vi "Rearrange images.vi"() -> ()   [LabVIEW 2015]
panel:
  in  "Selet tab":enum16{"Diagnostics", "Main"}(ring)
  in  "Type of label":u16(ring) items=["Combo", "String"]
  in  "Update\nTables":bool=TRUE
  in  "#Racks":u8
  in  "Camera names":string[](array[string])
  in  "Table column headers":string[](array[string])
  in  "Image indicator layouts 2":T1(array[cluster])=[{"NumberOfImageIndicators"=0.0, "ImageSpecificData"=[{"Width"=0.0, "Left"=0.0, "Top"=0.0, "Image Percentage"={"Height"=0.0, "Width correction"=0.0, "Height correction"=0.0, "Left correction"=0.0, "Top correction"=0.0}, "String Percentage"={"Height"=0.0, "Width correction"=0.0, "Height correction"=0.0, "Left correction"=0.0, "Top correction"=0.0}}, {"Width"=0.0, "Left"=0.0, "Top"=0.0, "Image Percentage"={"Height"=0.0, "Width correction"=0.0, "Height correction"=0.0, "Left correction"=0.0, "Top correction"=0.0}, "String Percentage"={"Height"=0.0, "Width correction"=0.0, "Height correction"=0.0, "Left correction"=0.0, "Top correction"=0.0}}, {"Width"=0.5, "Left"=0.0, "Top"=0.0, "Image Percentage"={"Height"=0.45, "Width correction"=-10.0, "Height correction"=0.0, "Left correction"=0.0, "Top correction"=0.0}, "String Percentage"={"Height"=0.05, "Width correction"=-5.0, "Height correction"=0.0, "Left correction"=0.0, "Top correction"=0.0}}, {"Width"=0.5, "Left"=0.0, "Top"=0.5, "Image Percentage"={"Height"=0.0, "Width correction"=-10.0, "Height correction"=0.0, "Left correction"=0.0, "Top correction"=0.0}, "String Percentage"={"Height"=0.0, "Width correction"=-5.0, "Height correction"=0.0, "Left correction"=0.0, "Top correction"=0.0}}, {"Width"=0.5, "Left"=0.5, "Top"=0.0, "Image Percentage"={"Height"=0.95, "Width correction"=-10.0, "Height correction"=0.0, "Left correction"=0.0, "Top correction"=0.0}, "String Percentage"={"Height"=0.05, "Width correction"=-5.0, "Height correction"=0.0, "Left correction"=0.0, "Top correction"=0.0}}]}, {"NumberOfImageIndicators"=0.0, "ImageSpecificData"=[]}, {"NumberOfImageIndicators"=0.0, "ImageSpecificData"=[{"Width"=0.5, "Left"=0.0, "Top"=0.0, "Image Percentage"={"Height"=0.45, "Width correction"=-7.0, "Height correction"=0.0, "Left correction"=0.0, "Top correction"=0.0}, "String Percentage"={"Height"=0.05, "Width correction"=-5.0, "Height correction"=0.0, "Left correction"=0.0, "Top correction"=0.0}}, {"Width"=0.5, "Left"=0.0, "Top"=0.5, "Image Percentage"={"Height"=0.45, "Width correction"=-7.0, "Height correction"=0.0, "Left correction"=0.0, "Top correction"=0.0}, "String Percentage"={"Height"=0.05, "Width correction"=-5.0, "Height correction"=0.0, "Left correction"=0.0, "Top correction"=0.0}}, {"Width"=0.5, "Left"=0.5, "Top"=0.0, "Image Percentage"={"Height"=0.95, "Width correction"=-7.0, "Height correction"=0.0, "Left correction"=0.0, "Top correction"=0.0}, "String Percentage"={"Height"=0.05, "Width correction"=-5.0, "Height correction"=0.0, "Left correction"=0.0, "Top correction"=0.0}}, {"Width"=0.5, "Left"=0.0, "Top"=0.5, "Image Percentage"={"Height"=0.45, "Width correction"=-7.0, "Height correction"=0.0, "Left correction"=0.0, "Top correction"=0.0}, "String Percentage"={"Height"=0.05, "Width correction"=-5.0, "Height correction"=0.0, "Left correction"=0.0, "Top correction"=0.0}}, {"Width"=0.5, "Left"=0.5, "Top"=0.0, "Image Percentage"={"Height"=0.0, "Width correction"=-7.0, "Height correction"=0.0, "Left correction"=0.0, "Top correction"=0.0}, "String Percentage"={"Height"=0.0, "Width correction"=-5.0, "Height correction"=0.0, "Left correction"=0.0, "Top correction"=0.0}}]}]
  in  "References":T2
  out "error out":errorcluster
  in  "error in (no error)":errorcluster
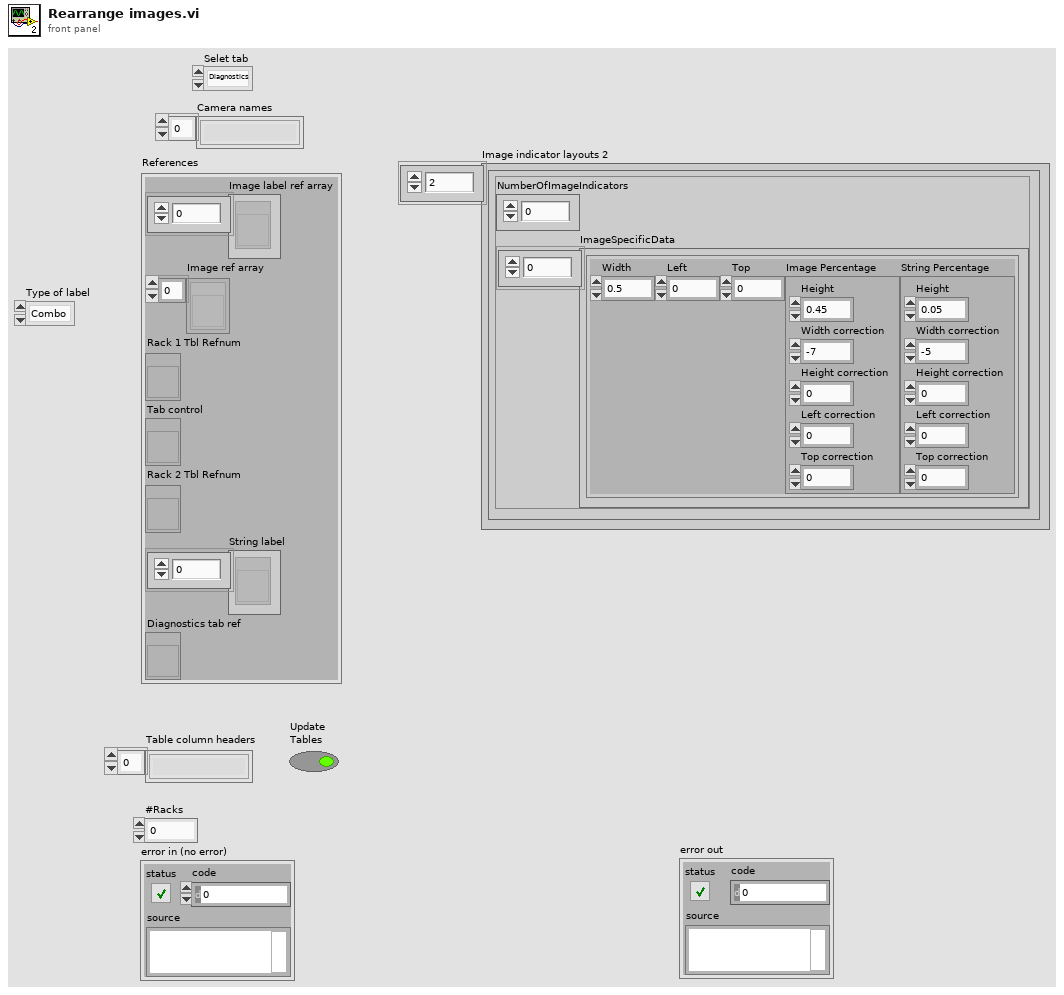
[diagram p1: front panel]
types:
  T1 = cluster{"NumberOfImageIndicators":dbl, "ImageSpecificData":cluster{"Width":dbl, "Left":dbl, "Top":dbl, "Image Percentage":cluster{"Height":dbl, "Width correction":dbl, "Height correction":dbl, "Left correction":dbl, "Top correction":dbl}, "String Percentage":cluster{"Height":dbl, "Width correction":dbl, "Height correction":dbl, "Left correction":dbl, "Top correction":dbl}}[]}[]
  T2 = cluster{"Image label ref array":refnum<vi>[], "Image ref array":refnum<vi>[], "Rack 1 Tbl Refnum":refnum<vi>, "Tab control":refnum<vi>, "Rack 2 Tbl Refnum":refnum<vi>, "String label":refnum<vi>[], "Diagnostics tab ref":refnum<vi>}
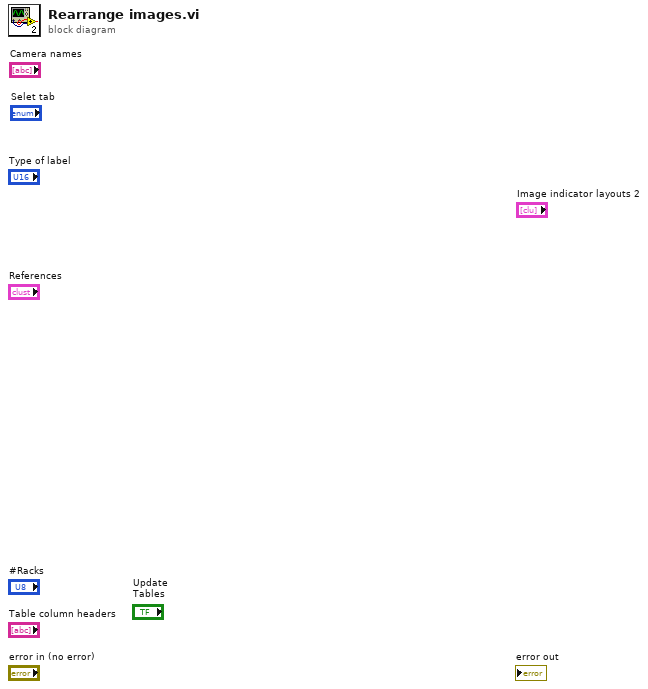
[diagram p0: block diagram]
diagram:
